vi "Unbenannt 2.vi"() -> ()   [LabVIEW 2010]
uses:
  <vilib>/Instr/_visa.llb/VISA Configure Serial Port (Instr).vi
  <vilib>/rvi/interface/nirviOpenFPGA/nirviOpenFPGA.xnode
  C:/Users/HAGAR-IV/Desktop/Zeugs/Johnny/pertrasgc fpga/fpga-programm.vi
  <vilib>/userDefined/High Color/nirio_resource_hc.ctl
  <vilib>/rvi/interface/nirviReadWriteControl/nirviReadWriteControl.xnode
  <vilib>/rvi/errors/niLvFpgaWhatHappensToTopLevelVI.ctl
  <vilib>/rvi/interface/common/niFpgaNodeNameForErrorReporting.ctl
  <vilib>/rvi/errors/niLvFpgaAdjustHostInterfaceError.vi
  <vilib>/rvi/interface/nirviCloseFPGA/nirviCloseFPGA.xnode
  <vilib>/RVI Host/nirviSupport.llb/nirviErrorClusterFromErrorCode.vi
  <vilib>/FPGAPlugInAG/cRIO-9114/niLvFpga_Close_cRIO-9114.vi
panel:
  out "Mod1/AIs.I/O Item":fxp<+/-,26,5> format="%.23g"
  in  "Stopp":bool
  out "Lesepuffer":string
  in  "VISA resource name":refnum<visa-resource-name> caption="VISA-Ressourcenname"
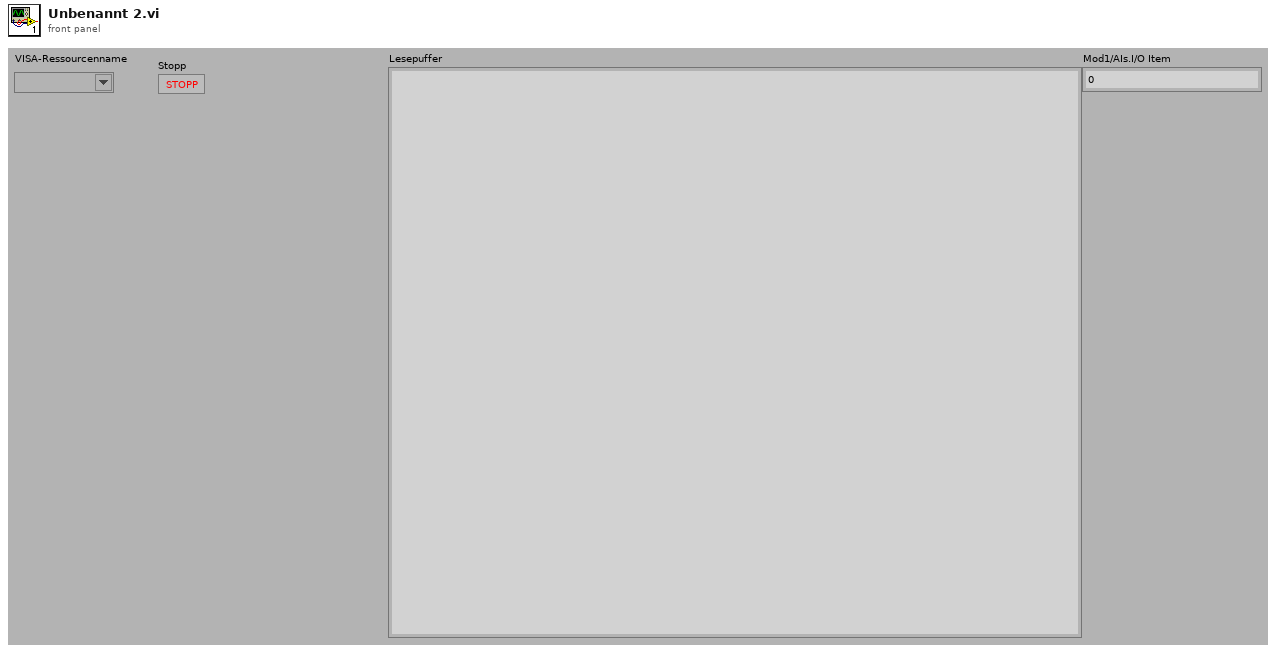
[diagram p1: front panel]
types:
  T1 = typedef "niFpgaNodeNameForErrorReporting.ctl" = enum16{"Open FPGA VI Reference", "Read/Write Control", "Invoke Method: Abort", "Invoke Method: Acknowledge IRQ", "Invoke Method: Download", "Invoke Method: FIFO.Configure", "Invoke Method: FIFO.Read", "Invoke Method: FIFO.Start", "Invoke Method: FIFO.Stop", "Invoke Method: FIFO.Write", "Invoke Method: Reset", "Invoke Method: Run", "Invoke Method: Wait on IRQ", "Close FPGA VI Reference"}
  T2 = typedef "niLvFpgaWhatHappensToTopLevelVI.ctl" = enum16{"top level VI scripted behind XNode", "top level VI inlined behind XNode"}
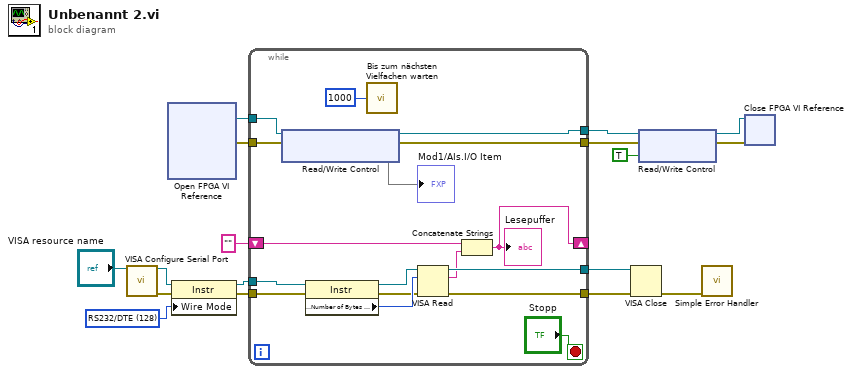
[diagram p0: block diagram]
diagram:
  w12 = i16 128 items=["Unknown"=-1, "RS485/Wire4"=0, "RS485/Wire2-EchoDTR"=1, "RS485/Wire2-CtrlDTR"=2, "RS485/Wire2-Auto"=3, "RS232/DTE"=128, "RS232/DCE"=129, "RS232/AUTO"=130] ("Serial Settings:Wire Mode")
  n1 = call-poly "VISA Configure Serial Port"("VISA resource name"="VISA resource name") -> ("VISA resource name out"=w16:refnum<visa-resource-name>, "error out"=w15:errorcluster)  [unwired: 13 in]
  n2 = xnode "Open FPGA VI Reference"() -> ("FPGA VI Reference Out"=w7:refnum<k20>, "error out"=w3:errorcluster)  [unwired: 2 in]
  n3 = property class="Instr"(reference=w16, error in=w15, "Wire Mode"=w12) -> (reference out=w14:refnum<visa-resource-name>, error out=w13:errorcluster)
  n4 = while {
    tunnel: w14 -> [w31]
    tunnel: w13 -> [w30]
    tunnel: [w29] -> w11
    tunnel: [w28] -> w10
    shift-right: [w23] -> _
    shift-left: "" -> [w24]
    tunnel: w7 -> [w22]
    tunnel: [w20] -> w6
    tunnel: w3 -> [w19]
    tunnel: [w18] -> w2
    stop <- "Stopp" stop-if-true
    n5 = xnode "Read/Write Control"("FPGA VI Reference In"=w22, "error in"=w19) -> ("FPGA VI Reference Out"=w20:refnum<k20>, "error out"=w18:errorcluster, "Mod1/AIs.I/O Item"=→"Mod1/AIs.I/O Item")
    n6 = property class="Instr"(reference=w31, error in=w30) -> (reference out=w34:refnum<visa-resource-name>, error out=w32:errorcluster, "Serial Settings:Number of Bytes at Serial Port"=w33:u32)
    n7 = call "Bis zum nächsten Vielfachen warten"("Count(mSec)"=u32 1000) -> ()  [unwired: 1 out]
    n8 = VISA Read(VISA resource name=w34, byte count=w33, error in (no error)=w32) -> (VISA resource name out=w29:refnum<visa-resource-name>, read buffer=w25:string, error out=w28:errorcluster)  [unwired: 1 out]
    n9 = Concatenate Strings(w24, w25) -> (w23:string)
    "Lesepuffer" <- w23
  }
  n10 = VISA Close(VISA resource name=w11, error in (no error)=w10) -> (error out=w9:errorcluster)
  n11 = xnode "Read/Write Control"("FPGA VI Reference In"=w6, "error in"=w2, "global stop"=TRUE) -> ("FPGA VI Reference Out"=w4:refnum<k20>, "error out"=w1:errorcluster)
  n12 = call <vilib>:"Simple Error Handler.vi"("error in (no error)"=w9) -> ()  [unwired: 4 in, 5 out]
  n13 = xnode "Close FPGA VI Reference"("FPGA VI Reference In"=w4, "error in"=w1) -> ()  [unwired: 1 out]
